vi "Main_RT.vi"() -> ()   [LabVIEW 2013]
uses:
  <vilib>/rvi/interface/nirviOpenFPGA/nirviOpenFPGA.xnode
  <vilib>/rvi/interface/nirviMethod/nirviMethod.xnode
  <vilib>/FPGAPlugInAG/Dynamic/niLvFpga_Reset_Dynamic.vi
  <vilib>/FPGAPlugInAG/Dynamic/niLvFpga_Run_Dynamic.vi
  <vilib>/rvi/interface/nirviCloseFPGA/nirviCloseFPGA.xnode
  <vilib>/FPGAPlugInAG/Dynamic/niLvFpga_Abort_Dynamic.vi
  <vilib>/rvi/interface/nirviReadWriteControl/nirviReadWriteControl.xnode
  NiFpgaLv.dll
  <vilib>/Utility/error.llb/Error Cluster From Error Code.vi
  <vilib>/rvi/interface/Simulation/niFpgaSimulationCallBeginRW.vi
  <vilib>/rvi/errors/niLvFpgaAdjustHostInterfaceError.vi
  <vilib>/ptbypt/NI_PtbyPt.lvlib
  <vilib>/Analysis/NI_AALBase.lvlib
  <vilib>/Analysis/1siggen.llb/Ramp Pattern by Samples.vi
  <vilib>/FPGAPlugInAG/Dynamic/niLvFpga_Close_Dynamic.vi
  FPGA Bitfiles/AKZ1_FPGATarget_MainFPGA_5-mRwLgXNqo.lvbitx
  AKZ 29082016/Main_FPGA.vi
  <vilib>/FPGAPlugInAG/cRIO-9082/niLvFpga_Open_cRIO-9082.vi
  <vilib>/rvi/interface/common/dynamic/niFpgaDynamicAddResources.vi
panel:
  in  "PID gains Fahrhebelsteller":T1={"proportional gain (Kc)"=1.5, "integral gain (Kc*Ts/Ti)"=0.1015625, "derivative gain (Kc*Td/Ts)"=0.0}
  in  "PID gains Bremse H":T1={"proportional gain (Kc)"=5.0, "integral gain (Kc*Ts/Ti)"=0.1015625, "derivative gain (Kc*Td/Ts)"=0.0}
  in  "PID gains Bremse R":T1={"proportional gain (Kc)"=5.0, "integral gain (Kc*Ts/Ti)"=0.1015625, "derivative gain (Kc*Td/Ts)"=0.0}
  in  "PID gains Bremse L":T1={"proportional gain (Kc)"=5.0, "integral gain (Kc*Ts/Ti)"=0.1015625, "derivative gain (Kc*Td/Ts)"=0.0}
  in  "Stop":bool
  out "Masteralarm":bool
  in  "Masteralarm On":bool
  in  "Alarme On":T2
  out "Alarme":T3
  in  "Systemreset / ON":bool
  in  "Tab Control":enum32{"H", "L-R", "H-L-R", "System"}(tab)
  out "Wellendrehmoment mit Übersetzung  H":dbl(knob) scale=-2000.0..2000.0
  out "Drehmoment Hinten":dbl(knob) scale=-2000.0..2000.0
  out "Drehzahl Hinten":dbl(knob) scale=0.0..3000.0
  in  "Bremse\nFrei H":bool
  in  "Richtung H\nRückwärts":bool
  in  "Reset / On\n H":bool
  in  "Steuerung\nOn H":bool
  in  "Lüftung\nOn H":bool
  out "Meldungen H":T4
  in  "Wellendrehzahl\n Soll H":dbl(slide) scale=0.0..3000.0
  out "Wellendrehzahl mit Übersetzung H":dbl(knob) scale=0.0..12000.0
  in  "Übersetzung H":dbl=1.0
  in  "sample length H":i32=1000
  out "Abweichung":dbl(knob) scale=-30.0..30.0
  in  "Wellen\nmoment\n Soll":dbl(slide) scale=0.0..2000.0
  in  "Drehzahl/moment LR":bool
  out "Wellendrehmoment mit Übersetzung":dbl(knob) scale=-400.0..400.0
  out "Drehmoment Rechts":dbl(knob) scale=-2000.0..2000.0
  out "Drehmoment Links":dbl(knob) scale=-2000.0..2000.0
  out "Drehzahl Rechts":dbl(knob) scale=0.0..2000.0
  out "Drehzahl Links":dbl(knob) scale=0.0..2000.0
  in  "Bremse\nFrei":bool
  in  "Richtung\nRückwärts":bool
  in  "Reset / On":bool
  in  "Steuerung\nOn":bool
  in  "Lüftung\nOn":bool
  out "Meldungen L-R":T5
  in  "Wellen\ndrehzahl\n Soll":dbl(slide) scale=0.0..2000.0
  out "Wellendrehzahl mit Übersetzung":dbl(knob) scale=0.0..5000.0
  in  "Übersetzung":dbl=4.55
  in  "sample length LR":i32=1000
  in  "Count (mSec)":u32=10
  in  "Rampe Start":bool
  in  "Rampe Up":bool
  in  "Rampe Stop":bool
  out "Rampe Aktiv":bool
  in  "samples":i32=6000
  in  "end":dbl=1055.0 format="%0.2f"
  in  "start":dbl=192.0 format="%0.2f"
  in  "type":u16(ring) items=["Linear", "Logarithmic"]
  in  "Rampe \nmilliseconds to wait":u32=10
  out "output L":dbl format="%.2f"
  in  "Count Rampe (mSec)":u32=2
  in  "sample length DM":i32=1000
  in  "Tab Control 2":enum32{"Benzinmotor", "Elektromototr"}(tab)
  in  "Fahrregler Up":bool
  out "output F":dbl
  in  "Fahrregler Stop":bool
  out "Fahrregler Aktiv":bool
  in  "Fahrregler Start":bool
  in  "Regler":bool
  in  "Freigabe":bool
  in  "Wait":bool
  in  "Kühlung Soll":dbl(slide) scale=0.0..100.0
  out "Kühlwasser":u8(slide) scale=0.0..100.0
  in  "Motor\nStart":bool
  in  "Vorglühen\nOn":bool
  in  "Zündung\nOn":bool
  in  "Kraftstoff\nOn":bool
  out "Fahrhebelsteller":u8(slide) scale=0.0..100.0
  in  "Fahrhebelsteller Soll":dbl(slide) scale=0.0..100.0
  in  "Freigabe":bool
  in  "Kupplung\nOffen":bool
  out "Kupplung":cluster{"Offen":bool, "Geschlossen":bool}
  in  "type 2":u16(ring) items=["Linear", "Logarithmic"]
  in  "samples 2":i32=3000
  in  "end 2":dbl=100.0 format="%0.2f"
  in  "start 2":dbl format="%0.2f"
  in  "Fahrregler milliseconds to wait":u32=10
  out "Wellenmoment ohne":dbl
  in  "Count (mSec) Fahrhebel":u32=10
  out "Höhe M":fxp<+/-,24,5> format="%#.2g"
  out "Endlage Unten M":bool
  out "Endlage Oben M":bool
  out "Oben M":bool
  out "Unten M":bool
  in  "Freigabe Höhe M":bool
  in  "Richtung Höhe M":bool
  in  "Freigabe Drehzahl M":bool
  in  "Richtung Drehzahl M":bool
  in  "Freigabe Bremse M":bool
  in  "Run Button":bool
  in  "Hydraulikpumpensteller":dbl=11.0
  in  "Manual":bool
  in  "Up Button":bool
  in  "Down Button":bool
  in  "RPMK":dbl=300.0
  out "Step 1":bool
  out "Step 3":bool
  in  "Höhe":dbl=8.3
  in  "Zeit Rampe":i32=150
  out "Step 4":bool
  in  "DOWN":bool
  out "Step 5":bool
  in  "Zeit Down":i32=300
  out "Step 6":bool
  out "Step 7":bool
  out "Step 8":bool
  in  "RAMPE":bool
  in  "Drehmoment Motor":dbl
  in  "milliseconds to wait":u32=10000
  in  "Hydraulikkupplung":dbl
  # "Vorwärts"
  # "Vorwärts"
  # "Links"
  # "Rechts"
  # "System nicht bereit!"
  # "Geschlossen"
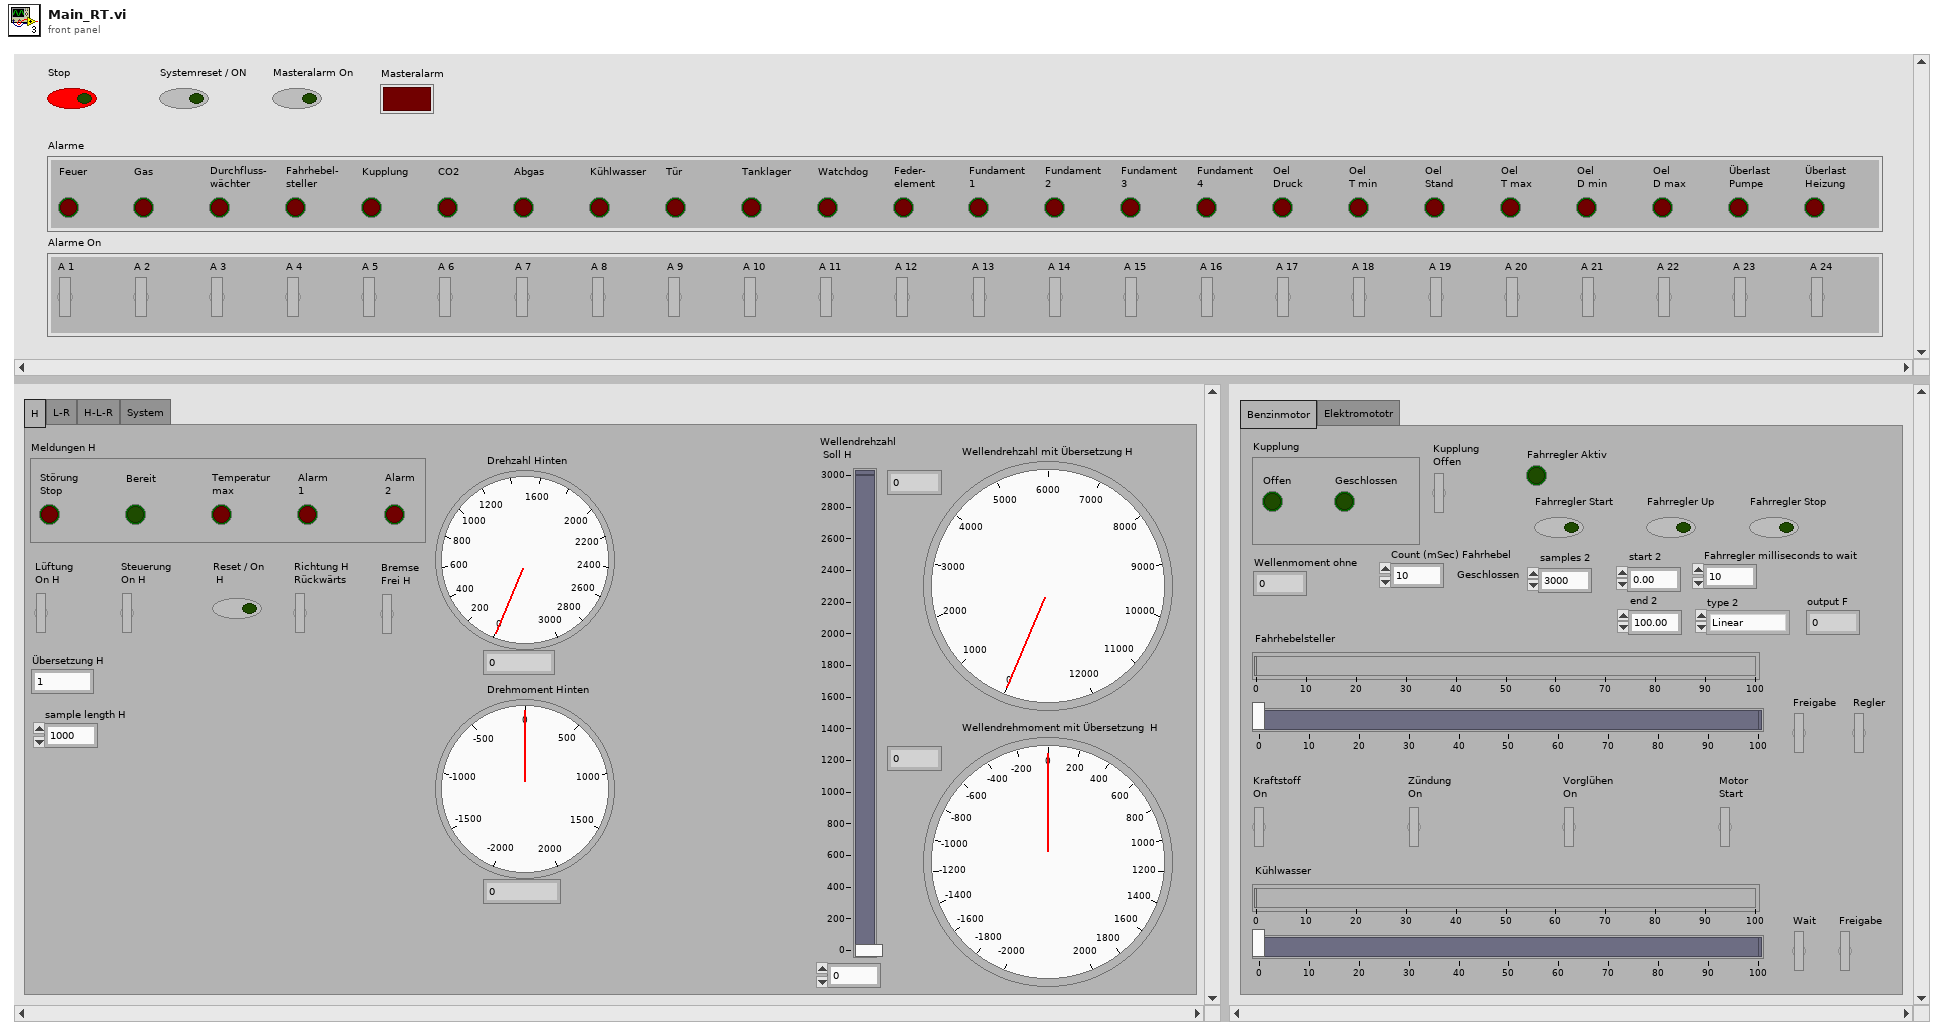
[diagram p1: front panel]
types:
  T1 = cluster{"proportional gain (Kc)":fxp<+/-,16,8>, "integral gain (Kc*Ts/Ti)":fxp<+/-,16,8>, "derivative gain (Kc*Td/Ts)":fxp<+/-,16,8>}
  T2 = cluster{"A 1":bool, "A 2":bool, "A 3":bool, "A 4":bool, "A 5":bool, "A 6":bool, "A 7":bool, "A 8":bool, "A 9":bool, "A 10":bool, "A 11":bool, "A 12":bool, "A 13":bool, "A 14":bool, "A 15":bool, "A 16":bool, "A 17":bool, "A 18":bool, "A 19":bool, "A 20":bool, "A 21":bool, "A 22":bool, "A 23":bool, "A 24":bool}
  T3 = cluster{"Feuer\n":bool, "Gas\n":bool, "Durchfluss-\nwächter":bool, "Fahrhebel-\nsteller":bool, "Kupplung\n":bool, "CO2\n":bool, "Abgas\n":bool, "Kühlwasser\n":bool, "Tür\n":bool, "Tanklager\n":bool, "Watchdog\n":bool, "Feder-\nelement":bool, "Fundament\n1":bool, "Fundament\n2":bool, "Fundament\n3":bool, "Fundament\n4":bool, "Oel\nDruck":bool, "Oel\nT min":bool, "Oel\nStand":bool, "Oel\nT max":bool, "Oel\nD min":bool, "Oel\nD max":bool, "Überlast\nPumpe":bool, "Überlast\nHeizung":bool}
  T4 = cluster{"Störung\nStop":bool, "Bereit\n":bool, "Temperatur\nmax":bool, "Alarm\n1":bool, "Alarm\n2":bool}
  T5 = cluster{"Störung\nStop":bool, "Bereit\n":bool, "Temperatur\nmax":bool, "Alarm\n1":bool, "Alarm\n2":bool, "Störung\nStop":bool, "Bereit\n":bool, "Temperatur\nmax":bool, "Alarm\n1":bool, "Alarm\n2":bool}
  T6 = cluster{"Mod5/Alarm 1 Feuer":bool, "Mod5/Alarm 2 Gas":bool, "Mod5/Alarm 3 Durchflusswächter":bool, "Mod5/Alarm 4 Fahrhebelsteller":bool, "Mod5/Alarm 5 Kupplung":bool, "Mod5/Alarm 6 CO2":bool, "Mod5/Alarm 7 Abgas":bool, "Mod5/Alarm 8 Kühlwasser":bool, "Mod5/Alarm 9 Tür":bool, "Mod5/Alarm 10 Tanklager":bool, "Mod5/Alarm 11 Watchdog":bool, "Mod5/Alarm 12 Federelement":bool, "Mod5/Alarm 13 Fundament 1":bool, "Mod5/Alarm 14 Fundament 2":bool, "Mod5/Alarm 15 Fundament 3":bool, "Mod5/Alarm 16 Fundament 4":bool, "Mod6/Alarm 17 Differnzdruck Öl":bool, "Mod6/Alarm 19 Temperatur Min ÖL":bool, "Mod6/Alarm 18 Nivau Öl":bool, "Mod6/Alarm 20 Temperatur Max Öl":bool, "Mod6/Alarm 21 Druck Min Öl":bool, "Mod6/Alarm 22 Druck Max Öl":bool, "Mod6/Alarm 23 Überlast Pumpe Öl":bool, "Mod6/Alarm 24 Überlast Heizung Öl":bool}
  T7 = cluster{"Mod5/Störung Bremse L":bool, "Mod5/Bereit Bremse L":bool, "Mod5/Temperatur Bremse L":bool, "Mod5/Alarm 1 Bremse L":bool, "Mod5/Alarm 2 Bremse L":bool, "Mod5/Störung Bremse R":bool, "Mod5/Bereit Bremse R":bool, "Mod5/Temperatur Bremse R":bool, "Mod5/Alarm 1 Bremse R":bool, "Mod5/Alarm 2 Bremse R":bool}
  T8 = cluster{"Mod6/Störung Bremse H":bool, "Mod6/Bereit Bremse H":bool, "Mod6/Temperatur Bremse H":bool, "Mod6/Alarm 1 Bremse H":bool, "Mod6/Alarm 2 Bremse H":bool}
  T9 = cluster{"Mod6/Kupplung Zu":bool, "Mod6/Kupplung Auf":bool}
diagram:
  n1 = while {
    stop <- "Stop" stop-if-true
    n2 = xnode "Open FPGA VI Reference"() -> ("FPGA VI Reference Out"=w8:refnum<k20>, "error out"=w7:errorcluster)  [unwired: 2 in]
    n3 = while {
      stop <- w14 stop-if-true
      n4 = case shown="True" "Rampe Start" {
        frame False {
        }
        frame True {
          n5 = flat-sequence {
            tunnel: ["samples"] -> w78
            tunnel: [w84] -> w76
            tunnel: [w83] -> w74
            tunnel: [w81] -> w72
            tunnel: "type" -> [w81]
            tunnel: [w104] -> w79
            tunnel: w78 -> [w104]
            tunnel: [w103] -> w77
            tunnel: w76 -> [w103]
            tunnel: [w102] -> w75
            tunnel: w74 -> [w102]
            tunnel: [w101] -> w73
            tunnel: w72 -> [w101]
            tunnel: w79 -> [w114]
            tunnel: w77 -> [w113]
            tunnel: w75 -> [w112]
            tunnel: w73 -> [w111]
            frame #0 {
              w80 = 300.0
              n6 = local write "Rampe Aktiv"(TRUE) -> ()
              n7 = Divide(x="end", y=w80) -> (x/y=w87:dbl)
              n8 = Divide(x="start", y=w80) -> (x/y=w84:dbl)
              n9 = call-poly <vilib>:"Ramp Pattern.vi"("type"=w81, "start"=w84, "end"=w87, "samples"="samples") -> ("Ramp Pattern"=w89:dbl[])  [unwired: 6 in, 1 out]
              n10 = Array Size(array=w89) -> (size(s)=w90:i32)
              n11 = while {
                tunnel: w89 -> [w100]
                tunnel: w90 -> [w99]
                tunnel: [w91] -> w83
                i -> [w96]
                stop <- w93 stop-if-true
                n12 = local read "Rampe Stop"() -> (w92:bool)
                n13 = Subtract(x=w99, y=1) -> (x-y=w97:i32)
                n14 = Equal?(x=w97, y=w96) -> (x = y?=w95:bool)
                n15 = Index Array(array=w100, index=w96) -> (element=w91:dbl)
                n16 = Or(x=w95, y=w92) -> (x .or. y?=w93:bool)
                n17 = local write "output L"(w91) -> ()
                n18 = Wait (ms)(milliseconds to wait="Rampe \nmilliseconds to wait") -> ()  [unwired: 1 out]
              }
            }
            frame #1 {
              n19 = while {
                stop <- w106 stop-if-true
                n20 = local read "Rampe Stop"() -> (w105:bool)
                n21 = Wait (ms)(milliseconds to wait=u32 100) -> ()  [unwired: 1 out]
                n22 = Or(x=w105, y="Rampe Up") -> (x .or. y?=w106:bool)
              }
            }
            frame #2 {
              n23 = call-poly <vilib>:"Ramp Pattern.vi"("type"=w111, "start"=w112, "end"=w113, "samples"=w114) -> ("Ramp Pattern"=w110:dbl[])  [unwired: 6 in, 1 out]
              n24 = Array Size(array=w110) -> (size(s)=w109:i32)
              n25 = while {
                tunnel: w110 -> [w124]
                tunnel: w109 -> [w123]
                i -> [w120]
                stop <- w117 stop-if-true
                n26 = Subtract(x=w123, y=1) -> (x-y=w121:i32)
                n27 = local read "Rampe Stop"() -> (w116:bool)
                n28 = Equal?(x=w121, y=w120) -> (x = y?=w118:bool)
                n29 = Index Array(array=w124, index=w120) -> (element=w115:dbl)
                n30 = Or(x=w118, y=w116) -> (x .or. y?=w117:bool)
                n31 = local write "output L"(w115) -> ()
                n32 = Wait (ms)(milliseconds to wait=u32 1) -> ()  [unwired: 1 out]
              }
            }
            frame #3 {
              w125 = FALSE
              n33 = local write "Rampe Start"(w125) -> ()
              n34 = local write "Rampe Aktiv"(w125) -> ()
              n35 = local write "Rampe Stop"(w125) -> ()
            }
          }
        }
      }
      n36 = case shown="True" "Fahrregler Start" {
        frame False {
        }
        frame True {
          n37 = flat-sequence {
            tunnel: "type 2" -> [w27]
            tunnel: ["samples 2"] -> w23
            tunnel: [w27] -> w21
            tunnel: [w26] -> w19
            tunnel: [w25] -> w17
            tunnel: w23 -> [w49]
            tunnel: [w49] -> w22
            tunnel: w21 -> [w48]
            tunnel: [w48] -> w20
            tunnel: w19 -> [w47]
            tunnel: [w47] -> w18
            tunnel: w17 -> [w46]
            tunnel: [w46] -> w16
            tunnel: w22 -> [w59]
            tunnel: w20 -> [w58]
            tunnel: w18 -> [w57]
            tunnel: w16 -> [w56]
            frame #0 {
              w32 = 10.0 ("y")
              n38 = local write "Fahrregler Aktiv"(TRUE) -> ()
              n39 = Divide(x="end 2", y=w32) -> (x/y=w34:dbl)
              n40 = Divide(x="start 2", y=w32) -> (x/y=w25:dbl)
              n41 = call-poly <vilib>:"Ramp Pattern.vi"("type"=w27, "start"=w25, "end"=w34, "samples"="samples 2") -> ("Ramp Pattern"=w30:dbl[])  [unwired: 6 in, 1 out]
              n42 = Array Size(array=w30) -> (size(s)=w29:i32)
              n43 = while {
                tunnel: w30 -> [w45]
                tunnel: w29 -> [w44]
                tunnel: [w36] -> w26
                i -> [w41]
                stop <- w39 stop-if-true
                n44 = local read "Fahrregler Stop"() -> (w38:bool)
                n45 = Index Array(array=w45, index=w41) -> (element=w36:dbl)
                n46 = Subtract(x=w44, y=1) -> (x-y=w42:i32)
                n47 = Equal?(x=w42, y=w41) -> (x = y?=w40:bool)
                n48 = local write "output F"(w36) -> ()
                n49 = Or(x=w40, y=w38) -> (x .or. y?=w39:bool)
                n50 = Wait (ms)(milliseconds to wait="Fahrregler milliseconds to wait") -> ()  [unwired: 1 out]
              }
            }
            frame #1 {
              n51 = while {
                stop <- w52 stop-if-true
                n52 = local read "Fahrregler Stop"() -> (w51:bool)
                n53 = Wait (ms)(milliseconds to wait=u32 100) -> ()  [unwired: 1 out]
                n54 = Or(x="Fahrregler Up", y=w51) -> (x .or. y?=w52:bool)
              }
            }
            frame #2 {
              n55 = call-poly <vilib>:"Ramp Pattern.vi"("type"=w58, "start"=w57, "end"=w56, "samples"=w59) -> ("Ramp Pattern"=w55:dbl[])  [unwired: 6 in, 1 out]
              n56 = Array Size(array=w55) -> (size(s)=w54:i32)
              n57 = while {
                tunnel: w55 -> [w69]
                tunnel: w54 -> [w68]
                i -> [w65]
                stop <- w63 stop-if-true
                n58 = local read "Fahrregler Stop"() -> (w62:bool)
                n59 = Index Array(array=w69, index=w65) -> (element=w61:dbl)
                n60 = Subtract(x=w68, y=1) -> (x-y=w66:i32)
                n61 = Equal?(x=w66, y=w65) -> (x = y?=w64:bool)
                n62 = local write "output F"(w61) -> ()
                n63 = Or(x=w64, y=w62) -> (x .or. y?=w63:bool)
                n64 = Wait (ms)(milliseconds to wait=u32 1) -> ()  [unwired: 1 out]
              }
            }
            frame #3 {
              w70 = FALSE
              n65 = local write "Fahrregler Aktiv"(w70) -> ()
              n66 = local write "Fahrregler Stop"(w70) -> ()
              n67 = local write "Fahrregler Start"(w70) -> ()
            }
          }
        }
      }
      n68 = local read "Stop"() -> (w14:bool)
    }
    n69 = xnode "Invoke Method"("FPGA VI Reference In"=w8, "error in"=w7) -> ("FPGA VI Reference Out"=w6:refnum<k20>, "error out"=w5:errorcluster)
    n70 = xnode "Invoke Method"("FPGA VI Reference In"=w6, "error in"=w5, "Wait Until Done (F)"=FALSE) -> ("FPGA VI Reference Out"=w1:refnum<k20>, "error out"=w12:errorcluster)
    n71 = while {
      tunnel: w1 -> [w415]
      tunnel: w12 -> [w414]
      tunnel: [w197] -> w11
      tunnel: [w244] -> w9
      stop <- w360 stop-if-true
      w151 = 0.0 ("f")
      w189 = 10.0
      w286 = 1800.0 ("y")
      w139 = fxp<+,24,5> 10.0 ("y")
      w131 = 200.0 ("y")
      w167 = 300.0 ("x")
      n72 = local read "Steuerung\nOn H"() -> (w211:bool)
      n73 = local read "Steuerung\nOn"() -> (w210:bool)
      n74 = Less?(x="Hydraulikpumpensteller", y=5.0) -> (x < y?=w193:bool)
      n75 = Select(t="RPMK", s="Down Button", f=0.0) -> (s? t:f=w277:dbl)
      n76 = local read "Stop"() -> (w360:bool)
      n77 = Negate(x=w277) -> (-x=w275:dbl)
      n78 = Select(t=5.0, s=w193, f="Hydraulikpumpensteller") -> (s? t:f=w190:dbl)
      n79 = Greater?(x="Drehmoment Motor", y=1000.0) -> (0:w257:bool)
      n80 = Or(x=w210, y=w211) -> (x .or. y?=w209:bool)
      n81 = feedback #1() -> (w319:bool)  [unwired: 1 in]
      n82 = Greater?(x=w190, y=50.0) -> (0:w269:bool)
      n83 = Greater?(x="Hydraulikkupplung", y=100.0) -> (0:w206:bool)
      n84 = xnode "Read/Write Control"("FPGA VI Reference In"=w415, "error in"=w414, "Mod3/Systemreset/ON"="Systemreset / ON", "stop"=w360, "Alarm On"="Masteralarm On", "Mod3/Blitzlicht"=w209, "Mod3/Horn"=w319, "PID gains Bremse L"="PID gains Bremse L", "PID gains Bremse R"="PID gains Bremse R", "PID gains Bremse H"="PID gains Bremse H", "PID gains"="PID gains Fahrhebelsteller") -> ("FPGA VI Reference Out"=w413:refnum<k20>, "error out"=w300:errorcluster, "Alarm"=w321:bool)
      "Masteralarm" <- w321
      n85 = Select(t="RPMK", s="Up Button", f=w275) -> (s? t:f=w274:dbl)
      n86 = Select(t=100.0, s=w206, f="Hydraulikkupplung") -> (s? t:f=w202:dbl)
      n87 = Select(t=1000.0, s=w257, f="Drehmoment Motor") -> (s? t:f=w254:dbl)
      n88 = Select(t=50.0, s=w269, f=w190) -> (s? t:f=w207:dbl)
      n89 = xnode "Read/Write Control"("FPGA VI Reference In"=w413, "error in"=w300) -> ("FPGA VI Reference Out"=w412:refnum<k20>, "error out"=w250:errorcluster, "Mod5/Alarm 1 Feuer"=w411:bool, "Mod5/Alarm 2 Gas"=w410:bool, "Mod5/Alarm 3 Durchflusswächter"=w408:bool, "Mod5/Alarm 4 Fahrhebelsteller"=w407:bool, "Mod5/Alarm 5 Kupplung"=w406:bool, "Mod5/Alarm 6 CO2"=w405:bool, "Mod5/Alarm 7 Abgas"=w404:bool, "Mod5/Alarm 8 Kühlwasser"=w403:bool, "Mod5/Alarm 9 Tür"=w402:bool, "Mod5/Alarm 10 Tanklager"=w401:bool, "Mod5/Alarm 11 Watchdog"=w400:bool, "Mod5/Alarm 12 Federelement"=w399:bool, "Mod5/Alarm 13 Fundament 1"=w398:bool, "Mod5/Alarm 14 Fundament 2"=w397:bool, "Mod5/Alarm 15 Fundament 3"=w396:bool, "Mod5/Alarm 16 Fundament 4"=w395:bool, "Mod6/Alarm 17 Differnzdruck Öl"=w394:bool, "Mod6/Alarm 19 Temperatur Min ÖL"=w393:bool, "Mod6/Alarm 18 Nivau Öl"=w392:bool, "Mod6/Alarm 20 Temperatur Max Öl"=w391:bool, "Mod6/Alarm 21 Druck Min Öl"=w390:bool, "Mod6/Alarm 22 Druck Max Öl"=w389:bool, "Mod6/Alarm 23 Überlast Pumpe Öl"=w388:bool, "Mod6/Alarm 24 Überlast Heizung Öl"=w387:bool)
      n90 = And(x="Masteralarm On", y=w321) -> (x .and. y?=w320:bool)
      n91 = feedback-in #1(w320) -> ()
      n92 = Select(t=w207, s="Run Button", f=0.0) -> (s? t:f=w282:dbl)
      n93 = Less Than 0?(x="Wellen\ndrehzahl\n Soll") -> (x < 0?=w243:bool)
      n94 = Divide(x=w274, y=345.0) -> (x/y=w272:dbl)
      n95 = Unbundle("Alarme On") -> ("A 1"=w384:bool, "A 2"=w383:bool, "A 3"=w382:bool, "A 4"=w381:bool, "A 5"=w380:bool, "A 6"=w379:bool, "A 7"=w378:bool, "A 8"=w377:bool, "A 9"=w376:bool, "A 10"=w375:bool, "A 11"=w374:bool, "A 12"=w373:bool, "A 13"=w372:bool, "A 14"=w371:bool, "A 15"=w370:bool, "A 16"=w369:bool, "A 17"=w368:bool, "A 18"=w367:bool, "A 19"=w366:bool, "A 20"=w365:bool, "A 21"=w364:bool, "A 22"=w363:bool, "A 23"=w362:bool, "A 24"=w361:bool)
      n96 = local read "Rampe Stop"() -> (w171:bool)
      n97 = local read "output L"() -> (w170:dbl)
      n98 = xnode "Read/Write Control"("FPGA VI Reference In"=w412, "error in"=w250, "Alarm 1 On"=w384, "Alarm 2 On"=w383, "Alarm 3 On"=w382, "Alarm 4 On"=w381, "Alarm 5 On"=w380, "Alarm 6 On"=w379, "Alarm 7 On"=w378, "Alarm 8 On"=w377, "Alarm 9 On"=w376, "Alarm 10 On"=w375, "Alarm 11 On"=w374, "Alarm 12 On"=w373, "Alarm 13 On"=w372, "Alarm 14 On"=w371, "Alarm 15 On"=w370, "Alarm 16 On"=w369, "Alarm 17 On"=w368, "Alarm 18 On"=w367, "Alarm 19 On"=w366, "Alarm 20 On"=w365, "Alarm 21 On"=w364, "Alarm 22 On"=w363, "Alarm 23 On"=w362, "Alarm 24 On"=w361) -> ("FPGA VI Reference Out"=w386:refnum<k20>, "error out"=w249:errorcluster)
      n99 = Bundle("Mod5/Alarm 1 Feuer"=w411, "Mod5/Alarm 2 Gas"=w410, "Mod5/Alarm 3 Durchflusswächter"=w408, "Mod5/Alarm 4 Fahrhebelsteller"=w407, "Mod5/Alarm 5 Kupplung"=w406, "Mod5/Alarm 6 CO2"=w405, "Mod5/Alarm 7 Abgas"=w404, "Mod5/Alarm 8 Kühlwasser"=w403, "Mod5/Alarm 9 Tür"=w402, "Mod5/Alarm 10 Tanklager"=w401, "Mod5/Alarm 11 Watchdog"=w400, "Mod5/Alarm 12 Federelement"=w399, "Mod5/Alarm 13 Fundament 1"=w398, "Mod5/Alarm 14 Fundament 2"=w397, "Mod5/Alarm 15 Fundament 3"=w396, "Mod5/Alarm 16 Fundament 4"=w395, "Mod6/Alarm 17 Differnzdruck Öl"=w394, "Mod6/Alarm 19 Temperatur Min ÖL"=w393, "Mod6/Alarm 18 Nivau Öl"=w392, "Mod6/Alarm 20 Temperatur Max Öl"=w391, "Mod6/Alarm 21 Druck Min Öl"=w390, "Mod6/Alarm 22 Druck Max Öl"=w389, "Mod6/Alarm 23 Überlast Pumpe Öl"=w388, "Mod6/Alarm 24 Überlast Heizung Öl"=w387) -> (→"Alarme":T6)  [unwired: 1 in]
      n100 = Multiply(x=w170, y=w167) -> (x*y=w168:dbl)
      n101 = Select(t=w202, s="Run Button", f=0.0) -> (s? t:f=w201:dbl)
      n102 = Select(t=w254, s="Run Button", f=0.0) -> (s? t:f=w253:dbl)
      n103 = Select(t=0.0, s=w243, f="Wellen\ndrehzahl\n Soll") -> (s? t:f=w169:dbl)
      n104 = Divide(x=w282, y=10.0) -> (x/y=w180:dbl)
      n105 = Select(t=w168, s=w171, f=w169) -> (s? t:f=w172:dbl)
      n106 = local read "Rampe Aktiv"() -> (w175:bool)
      n107 = local write "Wellen\ndrehzahl\n Soll"(w172) -> ()
      n108 = xnode "Read/Write Control"("FPGA VI Reference In"=w386, "error in"=w249) -> ("FPGA VI Reference Out"=w266:refnum<k20>, "error out"=w248:errorcluster, "Mod6/Anlage H-L-R"=w352:bool, "Mod6/Anlage H"=w359:bool, "Mod6/Anlage L-R"=w355:bool)
      n109 = Divide(x=w169, y=w167) -> (x/y=w178:dbl)
      n110 = Select(t=w272, s="Manual", f=0.0) -> (s? t:f=w267:dbl)
      n111 = Divide(x=w201, y=10.0) -> (x/y=w199:dbl)
      n112 = Divide(x=w253, y=100.0) -> (x/y=w251:dbl)
      n113 = Divide(x="Wellen\nmoment\n Soll", y=200.0) -> (x/y=w153:dbl)
      n114 = Select(t=w170, s=w175, f=w178) -> (s? t:f=w179:dbl)
      n115 = xnode "Read/Write Control"("FPGA VI Reference In"=w266, "error in"=w248, "Mod7/Hydraulikkupplung Soll"=w199, "Mod7/Hydraulikpumpensteller Soll"=w180, "Mod7/Höhe M Soll"=w267, "Mod4/Freigabe Höhe M"="Freigabe Höhe M", "Mod4/Richtung Höhe M"="Richtung Höhe M", "Mod4/Freigabe Drehzahl M"="Freigabe Drehzahl M", "Mod4/Richtung Drehzahl M"="Richtung Drehzahl M", "Mod4/Freigabe Bremse M"="Freigabe Bremse M", "Mod7/Drehmoment M Soll"=w251) -> ("FPGA VI Reference Out"=w299:refnum<k20>, "error out"=w247:errorcluster, "Mod8/Höhe M"=w288:fxp<+/-,24,5>, "Mod6/Endlage Oben M"=→"Endlage Oben M":bool, "Mod6/Oben M"=→"Oben M":bool, "Mod6/Unten M"=→"Unten M":bool, "Mod6/Endlage Unten M"=→"Endlage Unten M":bool)  [unwired: 2 out]
      n116 = Add(x=3900.0, y=w286) -> (x+y=w289:dbl)
      n117 = Select(t=w153, s="Drehzahl/moment LR", f=w179) -> (s? t:f=w186:dbl)
      n118 = Less Than 0?(x="Wellendrehzahl\n Soll H") -> (x < 0?=w234:bool)
      n119 = Select(t=2.0, s=w352, f=3.0) -> (s? t:f=w353:dbl)
      n120 = Negate(x=w186) -> (-x=w330:dbl)
      n121 = Select(t=0.0, s=w234, f="Wellendrehzahl\n Soll H") -> (s? t:f=w232:dbl)
      n122 = Select(t=1.0, s=w355, f=w353) -> (s? t:f=w356:dbl)
      n123 = xnode "Read/Write Control"("FPGA VI Reference In"=w299, "error in"=w247) -> ("FPGA VI Reference Out"=w349:refnum<k20>, "error out"=w246:errorcluster, "Mod5/Störung Bremse L"=w347:bool, "Mod5/Bereit Bremse L"=w346:bool, "Mod5/Temperatur Bremse L"=w345:bool, "Mod5/Alarm 1 Bremse L"=w344:bool, "Mod5/Alarm 2 Bremse L"=w343:bool, "Mod5/Störung Bremse R"=w342:bool, "Mod5/Bereit Bremse R"=w341:bool, "Mod5/Temperatur Bremse R"=w340:bool, "Mod5/Alarm 1 Bremse R"=w339:bool, "Mod5/Alarm 2 Bremse R"=w338:bool, "Mod6/Störung Bremse H"=w217:bool, "Mod6/Bereit Bremse H"=w216:bool, "Mod6/Temperatur Bremse H"=w215:bool, "Mod6/Alarm 1 Bremse H"=w214:bool, "Mod6/Alarm 2 Bremse H"=w213:bool)
      n124 = local read "Fahrregler Aktiv"() -> (w144:bool)
      n125 = local read "output F"() -> (w140:dbl)
      n126 = local read "Fahrregler Stop"() -> (w143:bool)
      n127 = Divide(x="Fahrhebelsteller Soll", y=w139) -> (x/y=w138:dbl)
      n128 = Divide(x="Kühlung Soll", y=w139) -> (x/y=w302:dbl)
      n129 = Multiply(x=w289, y=w288) -> (x*y=w287:dbl)
      n130 = Multiply(x=w140, y=w139) -> (x*y=w141:dbl)
      n131 = Select(t=0.0, s=w359, f=w356) -> (s? t:f=w358:dbl)
      n132 = Divide(x=w232, y=w167) -> (x/y=w230:dbl)
      n133 = Select(t=w141, s=w143, f="Fahrhebelsteller Soll") -> (s? t:f=w142:dbl)
      n134 = Select(t=w140, s=w144, f=w138) -> (s? t:f=w145:dbl)
      n135 = local write "Fahrhebelsteller Soll"(w142) -> ()
      n136 = property on="Tab Control" class="TabCtl (strict)"("Value"=w358) -> ()  [unwired: 2 in, 2 out]
      n137 = Bundle("Mod5/Störung Bremse L"=w347, "Mod5/Bereit Bremse L"=w346, "Mod5/Temperatur Bremse L"=w345, "Mod5/Alarm 1 Bremse L"=w344, "Mod5/Alarm 2 Bremse L"=w343, "Mod5/Störung Bremse R"=w342, "Mod5/Bereit Bremse R"=w341, "Mod5/Temperatur Bremse R"=w340, "Mod5/Alarm 1 Bremse R"=w339, "Mod5/Alarm 2 Bremse R"=w338) -> (→"Meldungen L-R":T7)  [unwired: 1 in]
      n138 = Divide(x=w287, y=w286) -> (x/y=w284:dbl)
      n139 = Select(t=w330, s="Richtung\nRückwärts", f=w186) -> (s? t:f=w182:dbl)
      n140 = Bundle("Mod6/Störung Bremse H"=w217, "Mod6/Bereit Bremse H"=w216, "Mod6/Temperatur Bremse H"=w215, "Mod6/Alarm 1 Bremse H"=w214, "Mod6/Alarm 2 Bremse H"=w213) -> (→"Meldungen H":T8)  [unwired: 1 in]
      n141 = Negate(x=w230) -> (-x=w229:dbl)
      n142 = call <vilib>:"Mean PtByPt.vi"("x"=w284, "sample length"=100) -> ("mean"=→"Höhe M":dbl)  [unwired: 2 in, 1 out]
      n143 = Select(t=w229, s="Richtung H\nRückwärts", f=w230) -> (s? t:f=w184:dbl)
      n144 = Select(t="Count Rampe (mSec)", s=w175, f="Count (mSec)") -> (s? t:f=w176:u32)
      n145 = Negate(x=w182) -> (-x=w183:dbl)
      n146 = Select(t=w153, s="Regler", f=w151) -> (s? t:f=w152:dbl)
      n147 = feedback #2() -> (w146:dbl)  [unwired: 1 in]
      n148 = Select(t=w146, s="Regler", f=w151) -> (s? t:f=w149:dbl)
      n149 = xnode "Read/Write Control"("FPGA VI Reference In"=w349, "error in"=w246, "Mod4/Kupplung"="Kupplung\nOffen", "Mod3/Fahrhebelsteller Freigabe"="Freigabe", "Fahrhebelsteller Soll (%)"=w145, "Mod3/Motor Vorglühen On"="Vorglühen\nOn", "Mod3/Motor Start"="Motor\nStart", "Mod3/Motor Zündung On"="Zündung\nOn", "Mod3/Kraftstoffpumpe On"="Kraftstoff\nOn", "Mod4/Temperaturregelung Off"="Wait", "Mod4/Temperaturregelung Freigabe"="Freigabe", "Kühlung Soll (°C)"=w302, "Regler Fahrhebelsteller"="Regler", "Vorgabe Fahrhebelsteller"=w152, "Ist Fahrhebelsteller"=w149, "Count (mSec) Fahrhebel"="Count (mSec) Fahrhebel") -> ("FPGA VI Reference Out"=w317:refnum<k20>, "error out"=w245:errorcluster, "Mod6/Kupplung Zu"=w315:bool, "Mod6/Kupplung Auf"=w314:bool, "Mod8/Fahrhebelsteller"=w301:fxp<+/-,24,5>)
      n150 = Multiply(x=w301, y=w189) -> (x*y=→"Fahrhebelsteller":dbl)
      n151 = Multiply(x=w301, y=w189) -> (x*y=→"Kühlwasser":dbl)
      n152 = Bundle("Mod6/Kupplung Zu"=w315, "Mod6/Kupplung Auf"=w314) -> (→"Kupplung":T9)  [unwired: 1 in]
      n153 = Reciprocal(x=2.0) -> (1/x=w328:dbl)
      n154 = feedback #3() -> (w263:dbl)  [unwired: 1 in]
      n155 = xnode "Read/Write Control"("FPGA VI Reference In"=w317, "error in"=w245, "Mod3/Steuerung On Bremse L"="Steuerung\nOn", "Mod3/Steuerungsreset Bremse L"="Reset / On", "Mod3/Bremsenfunktion On Bremse L"="Bremse\nFrei", "Mod3/Anlage On Bremse L"="Lüftung\nOn", "Mod3/Steuerung On Bremse R"="Steuerung\nOn", "Mod3/Steuerungsreset Bremse R"="Reset / On", "Mod3/Bremsenfunktion On Bremse R"="Bremse\nFrei", "Mod3/Anlage On Bremse R"="Lüftung\nOn", "Mod4/Steuerung On Bremse H"="Steuerung\nOn H", "Mod4/Steuerungsreset Bremse H"="Reset / On\n H", "Mod4/Bremsenfunktion On Bremse H"="Bremse\nFrei H", "Mod4/Anlage On Bremse H"="Lüftung\nOn H", "Vorgabe Bremse L"=w182, "Vorgabe Bremse R"=w183, "Vorgabe Bremse H"=w184, "Mod7/Out 1"=w263, "Drehzahl/moment LR"="Drehzahl/moment LR", "Count (mSec)"=w176) -> ("FPGA VI Reference Out"=w197:refnum<k20>, "error out"=w244:errorcluster, "Mod2/Drehzahl Bremse L"=w331:fxp<+/-,20,5>, "Mod2/Drehzahl Bremse R"=w333:fxp<+/-,20,5>, "Mod8/Drehmoment Bremse L"=w324:fxp<+/-,24,5>, "Mod8/Drehmoment Bremse  R"=w260:fxp<+/-,24,5>, "Mod2/Drehzahl Bremse H"=w228:fxp<+/-,20,5>, "Mod8/Drehmoment Bremse H"=w222:fxp<+/-,24,5>)
      n156 = Multiply(x=w324, y=w131) -> (x*y=w136:dbl)
      n157 = Multiply(x=w222, y=w131) -> (x*y=w223:dbl)
      n158 = Absolute Value(x=w331) -> (abs(x)=w332:fxp<+,20,5>)
      n159 = Absolute Value(x=w333) -> (abs(x)=w334:fxp<+,20,5>)
      n160 = Negate(x=w260) -> (-x=w323:fxp<+/-,25,6>)
      n161 = Absolute Value(x=w228) -> (abs(x)=w227:fxp<+,20,5>)
      n162 = Multiply(x=w167, y=w332) -> (x*y=w158:dbl)
      n163 = Multiply(x=w334, y=w167) -> (x*y=w157:dbl)
      n164 = Multiply(x=w323, y=w131) -> (x*y=w135:dbl)
      n165 = Multiply(x=w227, y=w167) -> (x*y=w226:dbl)
      n166 = call <vilib>:"Mean PtByPt.vi"("x"=w223, "sample length"="sample length H") -> ("mean"=w219:dbl)  [unwired: 2 in, 1 out]
      "Drehmoment Hinten" <- w219
      n167 = Divide(x=w219, y="Übersetzung H") -> (x/y=w221:dbl)
      n168 = call <vilib>:"Mean PtByPt.vi"("x"=w158, "sample length"="sample length LR") -> ("mean"=w156:dbl)  [unwired: 2 in, 1 out]
      "Drehzahl Links" <- w156
      n169 = call <vilib>:"Mean PtByPt.vi"("x"=w157, "sample length"="sample length LR") -> ("mean"=w155:dbl)  [unwired: 2 in, 1 out]
      "Drehzahl Rechts" <- w155
      n170 = call <vilib>:"Mean PtByPt.vi"("x"=w136, "sample length"="sample length DM") -> ("mean"=w162:dbl)  [unwired: 2 in, 1 out]
      "Drehmoment Links" <- w162
      n171 = call <vilib>:"Mean PtByPt.vi"("x"=w135, "sample length"="sample length DM") -> ("mean"=w161:dbl)  [unwired: 2 in, 1 out]
      "Drehmoment Rechts" <- w161
      n172 = call <vilib>:"Mean PtByPt.vi"("x"=w226, "sample length"="sample length H") -> ("mean"=w225:dbl)  [unwired: 2 in, 1 out]
      "Drehzahl Hinten" <- w225
      n173 = Add(x=w156, y=w155) -> (x+y=w329:dbl)
      n174 = Multiply(x=w225, y="Übersetzung H") -> (x*y=→"Wellendrehzahl mit Übersetzung H":dbl)
      n175 = Add(x=w162, y=w161) -> (x+y=w240:dbl)
      n176 = call <vilib>:"Mean PtByPt.vi"("x"=w221, "sample length"="sample length H") -> ("mean"=→"Wellendrehmoment mit Übersetzung  H":dbl)  [unwired: 2 in, 1 out]
      n177 = Add(x=w162, y=w161) -> (x+y=w130:dbl)
      n178 = Add(x=w136, y=w135) -> (x+y=w134:dbl)
      n179 = Divide(x=w130, y="Übersetzung") -> (x/y=w163:dbl)
      n180 = Subtract(x=w156, y=w155) -> (x-y=→"Abweichung":dbl)
      n181 = Divide(x=w240, y="Übersetzung") -> (x/y=→"Wellendrehmoment mit Übersetzung":dbl)
      n182 = Divide(x=w134, y="Übersetzung") -> (x/y=w132:dbl)
      n183 = Divide(x=w163, y=400.0) -> (x/y=w262:dbl)
      n184 = Multiply(x=w329, y=w328) -> (x*y=w326:dbl)
      n185 = Add(x=w262, y=5.0) -> (x+y=w129:dbl)
      n186 = call <vilib>:"Mean PtByPt.vi"("x"=w129, "sample length"="sample length DM") -> ("mean"=w128:dbl)  [unwired: 2 in, 1 out]
      n187 = Multiply(x=w326, y="Übersetzung") -> (x*y=→"Wellendrehzahl mit Übersetzung":dbl)
      n188 = feedback-in #3(w128) -> ()
      n189 = Divide(x=w132, y=w131) -> (x/y=w147:dbl)
      "Wellenmoment ohne" <- w147
      n190 = feedback-in #2(w147) -> ()
    }
    n191 = disable-structure shown="Disabled" {
      disable-tunnel: w1 -> [w417 _]
      frame Disabled {
        n192 = while {
          tunnel: w417 -> [w451]
          stop <- w452 stop-if-true
          n193 = local read "Höhe M"() -> (w426:fxp<+/-,24,5>)
          n194 = Subtract(x="Höhe", y=w426) -> (x-y=w448:dbl)
          n195 = Divide(x=w448, y=10.0) -> (x/y=w435:dbl)
          n196 = Add(x=w435, y=w426) -> (x+y=w447:dbl)
          n197 = Multiply(x=w435, y=2.0) -> (x*y=w445:dbl)
          n198 = Multiply(x=w435, y=3.0) -> (x*y=w442:dbl)
          n199 = Multiply(x=w435, y=4.0) -> (x*y=w439:dbl)
          n200 = Multiply(x=w435, y=5.0) -> (x*y=w436:dbl)
          n201 = Multiply(x=w435, y=6.0) -> (x*y=w427:dbl)
          n202 = Multiply(x=w435, y=7.0) -> (x*y=w428:dbl)
          n203 = Multiply(x=w435, y=8.0) -> (x*y=w429:dbl)
          n204 = Multiply(x=w435, y=9.0) -> (x*y=w430:dbl)
          n205 = Add(x=w445, y=w426) -> (x+y=w444:dbl)
          n206 = Add(x=w442, y=w426) -> (x+y=w441:dbl)
          n207 = Add(x=w439, y=w426) -> (x+y=w438:dbl)
          n208 = Add(x=w436, y=w426) -> (x+y=w425:dbl)
          n209 = Add(x=w427, y=w426) -> (x+y=w424:dbl)
          n210 = Add(x=w428, y=w426) -> (x+y=w423:dbl)
          n211 = Add(x=w429, y=w426) -> (x+y=w422:dbl)
          n212 = Add(x=w430, y=w426) -> (x+y=w419:dbl)
          n213 = case shown="True" "RAMPE" {
            tunnel: w451 -> [_ w510]
            tunnel: w447 -> [_ w504]
            tunnel: w444 -> [_ w503]
            tunnel: w441 -> [_ w498]
            tunnel: w438 -> [_ w493]
            tunnel: w425 -> [_ w473]
            tunnel: w424 -> [_ w472]
            tunnel: w423 -> [_ w471]
            tunnel: w422 -> [_ w470]
            tunnel: "Höhe" -> [_ w469]
            tunnel: "milliseconds to wait" -> [_ w468]
            tunnel: "milliseconds to wait" -> [_ w467]
            tunnel: "milliseconds to wait" -> [_ w466]
            tunnel: "milliseconds to wait" -> [_ w465]
            tunnel: "milliseconds to wait" -> [_ w464]
            tunnel: "milliseconds to wait" -> [_ w463]
            tunnel: "milliseconds to wait" -> [_ w462]
            tunnel: "milliseconds to wait" -> [_ w456]
            tunnel: w419 -> [_ w454]
            tunnel: "Zeit Rampe" -> [_ w453]
            frame False {
            }
            frame True {
              n214 = flat-sequence {
                tunnel: w510 -> [w516]
                tunnel: [w515] -> w509
                tunnel: [w523] -> w508
                tunnel: w509 -> [w522]
                tunnel: w504 -> [w521]
                tunnel: [w520] -> w506
                tunnel: w453 -> [w519]
                tunnel: w508 -> [w541]
                tunnel: [w541] -> w507
                tunnel: w506 -> [w540]
                tunnel: [w540] -> w505
                tunnel: w468 -> [w539]
                tunnel: w507 -> [w546]
                tunnel: [w545] -> w502
                tunnel: w505 -> [w544]
                tunnel: w503 -> [w543]
                tunnel: [w542] -> w500
                tunnel: w502 -> [w562]
                tunnel: [w562] -> w501
                tunnel: w500 -> [w561]
                tunnel: [w561] -> w499
                tunnel: w467 -> [w560]
                tunnel: w501 -> [w567]
                tunnel: [w566] -> w497
                tunnel: w499 -> [w565]
                tunnel: w498 -> [w564]
                tunnel: [w563] -> w495
                tunnel: w497 -> [w583]
                tunnel: [w583] -> w496
                tunnel: w495 -> [w582]
                tunnel: [w582] -> w494
                tunnel: w466 -> [w581]
                tunnel: w496 -> [w588]
                tunnel: [w587] -> w492
                tunnel: w494 -> [w586]
                tunnel: w493 -> [w585]
                tunnel: [w584] -> w482
                tunnel: w492 -> [w604]
                tunnel: [w604] -> w491
                tunnel: w482 -> [w603]
                tunnel: [w603] -> w481
                tunnel: w465 -> [w602]
                tunnel: w491 -> [w609]
                tunnel: [w608] -> w490
                tunnel: w481 -> [w607]
                tunnel: [w606] -> w480
                tunnel: w473 -> [w605]
                tunnel: w490 -> [w625]
                tunnel: [w625] -> w489
                tunnel: w480 -> [w624]
                tunnel: [w624] -> w479
                tunnel: w464 -> [w623]
                tunnel: w489 -> [w630]
                tunnel: [w629] -> w488
                tunnel: w479 -> [w628]
                tunnel: [w627] -> w478
                tunnel: w472 -> [w626]
                tunnel: w488 -> [w646]
                tunnel: [w646] -> w487
                tunnel: w478 -> [w645]
                tunnel: [w645] -> w477
                tunnel: w463 -> [w644]
                tunnel: w487 -> [w651]
                tunnel: [w650] -> w486
                tunnel: w477 -> [w649]
                tunnel: [w648] -> w476
                tunnel: w471 -> [w647]
                tunnel: w486 -> [w667]
                tunnel: [w667] -> w485
                tunnel: w476 -> [w666]
                tunnel: [w666] -> w475
                tunnel: w462 -> [w665]
                tunnel: w485 -> [w672]
                tunnel: [w671] -> w461
                tunnel: w475 -> [w670]
                tunnel: [w669] -> w460
                tunnel: w470 -> [w668]
                tunnel: w461 -> [w688]
                tunnel: [w688] -> w459
                tunnel: w460 -> [w687]
                tunnel: [w687] -> w457
                tunnel: w456 -> [w686]
                tunnel: w459 -> [w693]
                tunnel: [w692] -> w458
                tunnel: w457 -> [w691]
                tunnel: [w690] -> w455
                tunnel: w454 -> [w689]
                tunnel: w458 -> [w709]
                tunnel: [w709] -> w484
                tunnel: [w708] -> w474
                tunnel: w456 -> [w707]
                tunnel: w455 -> [w708]
                tunnel: w484 -> [w713]
                tunnel: [w712] -> w483
                tunnel: w474 -> [w711]
                tunnel: w469 -> [w710]
                tunnel: [w727] -> w513
                tunnel: w483 -> [w728]
                tunnel: w513 -> [w738]
                tunnel: [w737] -> w512
                tunnel: w512 -> [w757]
                tunnel: [w756] -> w511
                tunnel: w511 -> [w762]
                frame #0 {
                  w517 = FALSE
                  n215 = xnode "Read/Write Control"("FPGA VI Reference In"=w516, "Mod4/Freigabe Bremse M"=TRUE) -> ("FPGA VI Reference Out"=w515:refnum<k20>)  [unwired: 1 in, 1 out]
                  n216 = local write "Step 3"(w517) -> ()
                  n217 = local write "Step 4"(w517) -> ()
                  n218 = local write "Step 5"(w517) -> ()
                  n219 = local write "Step 6"(w517) -> ()
                  n220 = local write "Step 7"(w517) -> ()
                  n221 = local write "Step 8"(w517) -> ()
                  "Step 1" <- TRUE ("Boolean")
                }
                frame #1 {
                  n222 = while {
                    tunnel: w522 -> [w532]
                    tunnel: [w530] -> w523
                    tunnel: w521 -> [w527]
                    tunnel: [w526] -> w520
                    tunnel: w519 -> [w526]
                    stop <- w534 stop-if-true
                    n223 = local read "Höhe M"() -> (w528:fxp<+/-,24,5>)
                    n224 = Less Or Equal?(x=w528, y=w527) -> (x <= y?=w535:bool)
                    n225 = Divide(x=w526, y=345) -> (x/y=w537:dbl)
                    n226 = Not(x=w535) -> (.not. x?=w533:bool)
                    n227 = Select(t=w537, s=w535, f=0) -> (s? t:f=w531:dbl)
                    n228 = xnode "Read/Write Control"("FPGA VI Reference In"=w532, "Mod7/Höhe M Soll"=w531, "Mod4/Freigabe Bremse M"=FALSE) -> ("FPGA VI Reference Out"=w530:refnum<k20>)  [unwired: 1 in, 1 out]
                    n229 = Or(x=w533, y=w533) -> (x .or. y?=w534:bool)
                  }
                  n230 = local write "Step 1"(FALSE) -> ()
                  "Step 3" <- TRUE ("Boolean")
                }
                frame #2 {
                  n231 = Wait (ms)(milliseconds to wait=w539) -> ()  [unwired: 1 out]
                }
                frame #3 {
                  n232 = while {
                    tunnel: w546 -> [w553]
                    tunnel: [w551] -> w545
                    tunnel: w543 -> [w548]
                    tunnel: w544 -> [w547]
                    tunnel: [w547] -> w542
                    stop <- w555 stop-if-true
                    n233 = local read "Höhe M"() -> (w549:fxp<+/-,24,5>)
                    n234 = Less Or Equal?(x=w549, y=w548) -> (x <= y?=w556:bool)
                    n235 = Divide(x=w547, y=345) -> (x/y=w558:dbl)
                    n236 = Not(x=w556) -> (.not. x?=w554:bool)
                    n237 = Select(t=w558, s=w556, f=0) -> (s? t:f=w552:dbl)
                    n238 = xnode "Read/Write Control"("FPGA VI Reference In"=w553, "Mod7/Höhe M Soll"=w552, "Mod4/Freigabe Bremse M"=FALSE) -> ("FPGA VI Reference Out"=w551:refnum<k20>)  [unwired: 1 in, 1 out]
                    n239 = Or(x=w554, y=w554) -> (x .or. y?=w555:bool)
                  }
                }
                frame #4 {
                  n240 = Wait (ms)(milliseconds to wait=w560) -> ()  [unwired: 1 out]
                }
                frame #5 {
                  n241 = while {
                    tunnel: w567 -> [w574]
                    tunnel: [w572] -> w566
                    tunnel: w564 -> [w569]
                    tunnel: w565 -> [w568]
                    tunnel: [w568] -> w563
                    stop <- w576 stop-if-true
                    n242 = local read "Höhe M"() -> (w570:fxp<+/-,24,5>)
                    n243 = Less Or Equal?(x=w570, y=w569) -> (x <= y?=w577:bool)
                    n244 = Divide(x=w568, y=345) -> (x/y=w579:dbl)
                    n245 = Not(x=w577) -> (.not. x?=w575:bool)
                    n246 = Select(t=w579, s=w577, f=0) -> (s? t:f=w573:dbl)
                    n247 = xnode "Read/Write Control"("FPGA VI Reference In"=w574, "Mod7/Höhe M Soll"=w573, "Mod4/Freigabe Bremse M"=FALSE) -> ("FPGA VI Reference Out"=w572:refnum<k20>)  [unwired: 1 in, 1 out]
                    n248 = Or(x=w575, y=w575) -> (x .or. y?=w576:bool)
                  }
                }
                frame #6 {
                  n249 = Wait (ms)(milliseconds to wait=w581) -> ()  [unwired: 1 out]
                }
                frame #7 {
                  n250 = while {
                    tunnel: w588 -> [w595]
                    tunnel: [w593] -> w587
                    tunnel: w585 -> [w590]
                    tunnel: w586 -> [w589]
                    tunnel: [w589] -> w584
                    stop <- w597 stop-if-true
                    n251 = local read "Höhe M"() -> (w591:fxp<+/-,24,5>)
                    n252 = Less Or Equal?(x=w591, y=w590) -> (x <= y?=w598:bool)
                    n253 = Divide(x=w589, y=345) -> (x/y=w600:dbl)
                    n254 = Not(x=w598) -> (.not. x?=w596:bool)
                    n255 = Select(t=w600, s=w598, f=0) -> (s? t:f=w594:dbl)
                    n256 = xnode "Read/Write Control"("FPGA VI Reference In"=w595, "Mod7/Höhe M Soll"=w594, "Mod4/Freigabe Bremse M"=FALSE) -> ("FPGA VI Reference Out"=w593:refnum<k20>)  [unwired: 1 in, 1 out]
                    n257 = Or(x=w596, y=w596) -> (x .or. y?=w597:bool)
                  }
                }
                frame #8 {
                  n258 = Wait (ms)(milliseconds to wait=w602) -> ()  [unwired: 1 out]
                }
                frame #9 {
                  n259 = while {
                    tunnel: w609 -> [w616]
                    tunnel: [w614] -> w608
                    tunnel: w605 -> [w611]
                    tunnel: w607 -> [w610]
                    tunnel: [w610] -> w606
                    stop <- w618 stop-if-true
                    n260 = local read "Höhe M"() -> (w612:fxp<+/-,24,5>)
                    n261 = Less Or Equal?(x=w612, y=w611) -> (x <= y?=w619:bool)
                    n262 = Divide(x=w610, y=345) -> (x/y=w621:dbl)
                    n263 = Not(x=w619) -> (.not. x?=w617:bool)
                    n264 = Select(t=w621, s=w619, f=0) -> (s? t:f=w615:dbl)
                    n265 = xnode "Read/Write Control"("FPGA VI Reference In"=w616, "Mod7/Höhe M Soll"=w615, "Mod4/Freigabe Bremse M"=FALSE) -> ("FPGA VI Reference Out"=w614:refnum<k20>)  [unwired: 1 in, 1 out]
                    n266 = Or(x=w617, y=w617) -> (x .or. y?=w618:bool)
                  }
                }
                frame #10 {
                  n267 = Wait (ms)(milliseconds to wait=w623) -> ()  [unwired: 1 out]
                }
                frame #11 {
                  n268 = while {
                    tunnel: w630 -> [w637]
                    tunnel: [w635] -> w629
                    tunnel: w626 -> [w632]
                    tunnel: w628 -> [w631]
                    tunnel: [w631] -> w627
                    stop <- w639 stop-if-true
                    n269 = local read "Höhe M"() -> (w633:fxp<+/-,24,5>)
                    n270 = Less Or Equal?(x=w633, y=w632) -> (x <= y?=w640:bool)
                    n271 = Divide(x=w631, y=345) -> (x/y=w642:dbl)
                    n272 = Not(x=w640) -> (.not. x?=w638:bool)
                    n273 = Select(t=w642, s=w640, f=0) -> (s? t:f=w636:dbl)
                    n274 = xnode "Read/Write Control"("FPGA VI Reference In"=w637, "Mod7/Höhe M Soll"=w636, "Mod4/Freigabe Bremse M"=FALSE) -> ("FPGA VI Reference Out"=w635:refnum<k20>)  [unwired: 1 in, 1 out]
                    n275 = Or(x=w638, y=w638) -> (x .or. y?=w639:bool)
                  }
                }
                frame #12 {
                  n276 = Wait (ms)(milliseconds to wait=w644) -> ()  [unwired: 1 out]
                }
                frame #13 {
                  n277 = while {
                    tunnel: w651 -> [w658]
                    tunnel: [w656] -> w650
                    tunnel: w647 -> [w653]
                    tunnel: w649 -> [w652]
                    tunnel: [w652] -> w648
                    stop <- w660 stop-if-true
                    n278 = local read "Höhe M"() -> (w654:fxp<+/-,24,5>)
                    n279 = Less Or Equal?(x=w654, y=w653) -> (x <= y?=w661:bool)
                    n280 = Divide(x=w652, y=345) -> (x/y=w663:dbl)
                    n281 = Not(x=w661) -> (.not. x?=w659:bool)
                    n282 = Select(t=w663, s=w661, f=0) -> (s? t:f=w657:dbl)
                    n283 = xnode "Read/Write Control"("FPGA VI Reference In"=w658, "Mod7/Höhe M Soll"=w657, "Mod4/Freigabe Bremse M"=FALSE) -> ("FPGA VI Reference Out"=w656:refnum<k20>)  [unwired: 1 in, 1 out]
                    n284 = Or(x=w659, y=w659) -> (x .or. y?=w660:bool)
                  }
                }
                frame #14 {
                  n285 = Wait (ms)(milliseconds to wait=w665) -> ()  [unwired: 1 out]
                }
                frame #15 {
                  n286 = while {
                    tunnel: w672 -> [w679]
                    tunnel: [w677] -> w671
                    tunnel: w668 -> [w674]
                    tunnel: w670 -> [w673]
                    tunnel: [w673] -> w669
                    stop <- w681 stop-if-true
                    n287 = local read "Höhe M"() -> (w675:fxp<+/-,24,5>)
                    n288 = Less Or Equal?(x=w675, y=w674) -> (x <= y?=w682:bool)
                    n289 = Divide(x=w673, y=345) -> (x/y=w684:dbl)
                    n290 = Not(x=w682) -> (.not. x?=w680:bool)
                    n291 = Select(t=w684, s=w682, f=0) -> (s? t:f=w678:dbl)
                    n292 = xnode "Read/Write Control"("FPGA VI Reference In"=w679, "Mod7/Höhe M Soll"=w678, "Mod4/Freigabe Bremse M"=FALSE) -> ("FPGA VI Reference Out"=w677:refnum<k20>)  [unwired: 1 in, 1 out]
                    n293 = Or(x=w680, y=w680) -> (x .or. y?=w681:bool)
                  }
                }
                frame #16 {
                  n294 = Wait (ms)(milliseconds to wait=w686) -> ()  [unwired: 1 out]
                }
                frame #17 {
                  n295 = while {
                    tunnel: w693 -> [w700]
                    tunnel: [w698] -> w692
                    tunnel: w689 -> [w695]
                    tunnel: w691 -> [w694]
                    tunnel: [w694] -> w690
                    stop <- w702 stop-if-true
                    n296 = local read "Höhe M"() -> (w696:fxp<+/-,24,5>)
                    n297 = Less Or Equal?(x=w696, y=w695) -> (x <= y?=w703:bool)
                    n298 = Divide(x=w694, y=345) -> (x/y=w705:dbl)
                    n299 = Not(x=w703) -> (.not. x?=w701:bool)
                    n300 = Select(t=w705, s=w703, f=0) -> (s? t:f=w699:dbl)
                    n301 = xnode "Read/Write Control"("FPGA VI Reference In"=w700, "Mod7/Höhe M Soll"=w699, "Mod4/Freigabe Bremse M"=FALSE) -> ("FPGA VI Reference Out"=w698:refnum<k20>)  [unwired: 1 in, 1 out]
                    n302 = Or(x=w701, y=w701) -> (x .or. y?=w702:bool)
                  }
                }
                frame #18 {
                  n303 = Wait (ms)(milliseconds to wait=w707) -> ()  [unwired: 1 out]
                }
                frame #19 {
                  n304 = while {
                    tunnel: w713 -> [w720]
                    tunnel: [w718] -> w712
                    tunnel: w710 -> [w714]
                    tunnel: w711 -> [w715]
                    stop <- w722 stop-if-true
                    n305 = local read "Höhe M"() -> (w716:fxp<+/-,24,5>)
                    n306 = Less Or Equal?(x=w716, y=w714) -> (x <= y?=w723:bool)
                    n307 = Divide(x=w715, y=345) -> (x/y=w725:dbl)
                    n308 = Not(x=w723) -> (.not. x?=w721:bool)
                    n309 = Select(t=w725, s=w723, f=0) -> (s? t:f=w719:dbl)
                    n310 = xnode "Read/Write Control"("FPGA VI Reference In"=w720, "Mod7/Höhe M Soll"=w719, "Mod4/Freigabe Bremse M"=FALSE) -> ("FPGA VI Reference Out"=w718:refnum<k20>)  [unwired: 1 in, 1 out]
                    n311 = Or(x=w721, y=w721) -> (x .or. y?=w722:bool)
                  }
                }
                frame #20 {
                  n312 = while {
                    tunnel: w728 -> [w733]
                    tunnel: [w732] -> w727
                    stop <- "DOWN" stop-if-true
                    n313 = xnode "Read/Write Control"("FPGA VI Reference In"=w733, "Mod7/Höhe M Soll"=0.0 ("RPM KM"), "Mod4/Freigabe Bremse M"=TRUE) -> ("FPGA VI Reference Out"=w732:refnum<k20>)  [unwired: 1 in, 1 out]
                    n314 = Wait (ms)(milliseconds to wait=u32 1 ("Zu wartende ms")) -> ()  [unwired: 1 out]
                  }
                  n315 = local write "Step 3"(FALSE) -> ()
                  "Step 4" <- TRUE ("Boolean")
                }
                frame #21 {
                  n316 = while {
                    tunnel: w738 -> [w743]
                    tunnel: [w742] -> w737
                    stop <- w746 stop-if-true
                    n317 = local read "Höhe M"() -> (w748:fxp<+/-,24,5>)
                    n318 = Divide(x="Zeit Down", y=345) -> (x/y=w752:dbl)
                    n319 = Negate(x=w752) -> (-x=w747:dbl)
                    n320 = Greater Or Equal?(x=w748, y=3.8) -> (x >= y?=w749:bool)
                    n321 = Not(x=w749) -> (.not. x?=w745:bool)
                    n322 = Select(t=w747, s=w749, f=0) -> (s? t:f=w744:dbl)
                    n323 = xnode "Read/Write Control"("FPGA VI Reference In"=w743, "Mod7/Höhe M Soll"=w744, "Mod4/Freigabe Bremse M"=FALSE) -> ("FPGA VI Reference Out"=w742:refnum<k20>)  [unwired: 1 in, 1 out]
                    n324 = Or(x=w745, y=w745) -> (x .or. y?=w746:bool)
                  }
                  n325 = local write "Step 4"(FALSE) -> ()
                  "Step 5" <- TRUE ("Boolean")
                }
                frame #22 {
                  n326 = xnode "Read/Write Control"("FPGA VI Reference In"=w757, "Mod7/Höhe M Soll"=1.0 ("RPM KM"), "Mod4/Freigabe Bremse M"=TRUE) -> ("FPGA VI Reference Out"=w756:refnum<k20>)  [unwired: 1 in, 1 out]
                  n327 = local write "Step 5"(FALSE) -> ()
                  "Step 6" <- TRUE ("Boolean")
                }
                frame #23 {
                  n328 = local write "Step 6"(FALSE) -> ()
                  n329 = xnode "Read/Write Control"("FPGA VI Reference In"=w762, "Mod7/Höhe M Soll"=0.0 ("RPM KM"), "Mod4/Freigabe Bremse M"=TRUE) -> ()  [unwired: 1 in, 2 out]
                  "Step 7" <- TRUE ("Boolean")
                }
                frame #24 {
                  n330 = local write "RAMPE"(FALSE ("Play Button 2")) -> ()
                  n331 = local write "Step 7"(FALSE) -> ()
                  "Step 8" <- TRUE ("Boolean")
                }
              }
            }
          }
          n332 = local read "Stop"() -> (w452:bool)
        }
      }
      frame Enabled {
      }
    }
    n333 = xnode "Invoke Method"("FPGA VI Reference In"=w11, "error in"=w9) -> ("FPGA VI Reference Out"=w3:refnum<k20>, "error out"=w2:errorcluster)
    n334 = xnode "Close FPGA VI Reference"("FPGA VI Reference In"=w3, "error in"=w2) -> ()  [unwired: 1 out]
  }
